vi "Format Result Count Strings.vi"(11 "Results":T1) -> (3 "Array":string[][](array[string]))   [LabVIEW 2020, in "Execution UI.lvclass"]
uses:
  Execution UI.lvclass
  Framework/Result Model/Statistics.ctl
  Framework/Result Model/Result Model.lvclass
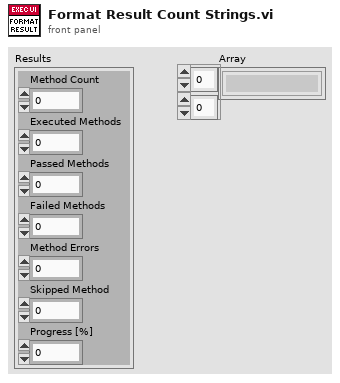
[diagram p1: front panel]
types:
  T1 = typedef "Result Model.lvclass/Statistics.ctl" = cluster{"Method Count":u32, "Executed Methods":u32, "Passed Methods":u32, "Failed Methods":u32, "Method Errors":u32, "Skipped Method":u32, "Progress [%]":dbl}
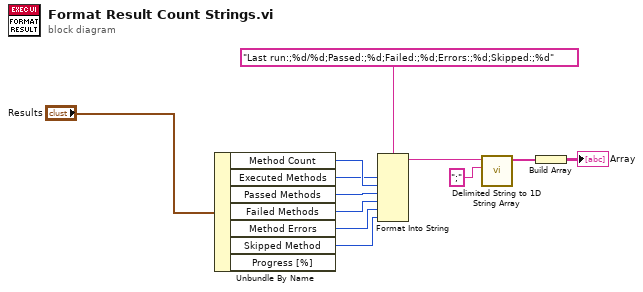
[diagram p0: block diagram]
diagram:
  n1 = Unbundle By Name("Results") -> ("Method Count"=w2:u32, "Executed Methods"=w1:u32, "Passed Methods"=w6:u32, "Failed Methods"=w7:u32, "Method Errors"=w9:u32, "Skipped Method"=w8:u32)  [unwired: 1 out]
  n2 = Format Into String(format string="Last run:;%d/%d;Passed:;%d;Failed:;%d;Errors:;%d;Skipped:;%d", w1, w2, w6, w7, w9, w8) -> (resulting string=w3:string)  [unwired: 2 in, 1 out]
  n3 = call <vilib>:"Delimited String to 1D String Array.vi"("delimiter"=";", "delimited string"=w3) -> ("string array"=w11:string[])  [unwired: 9 in]
  n4 = Build Array(w11) -> (→"Array":string[][])
